vi "Include_in_Preview.vi"(8 "error in (no error)":errorcluster, 11 "AB_Source_PackedItem in":refnum<class "AB_Source_PackedItem.lvclass">) -> (0 "error out":errorcluster, 2 "includeInPreview":bool)   [LabVIEW 2020, in "AB_Source_PackedItem.lvclass"]
uses:
  <vilib>/AppBuilder/AB_Classes/Source/PackedItem/AB_Source_PackedItem.lvclass
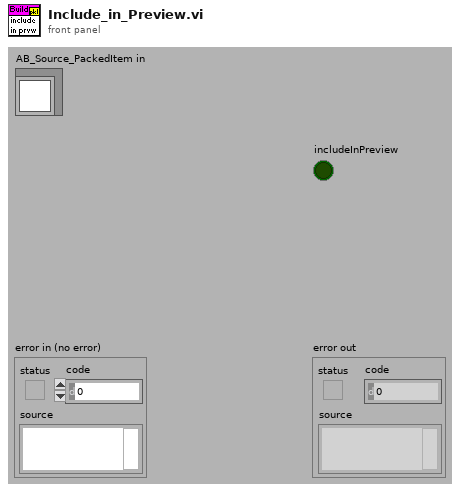
[diagram p1: front panel]
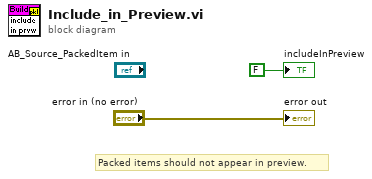
[diagram p0: block diagram]
diagram:
  # "Packed items should not appear in preview."
  "error out" <- "error in (no error)"
  "includeInPreview" <- FALSE ("includeInPreview")
